vi "Update status--Error.vi"(8 "error in (no error)":errorcluster, 10 "Remove call chain? [Default = False]":bool, 11 "Error message":string) -> (0 "error out":errorcluster)   [LabVIEW 2020, in "status_text_indicator.lvlib"]
uses:
  Status_Text_Indicator.lvlib
  PTRL/String_Control/string_control.lvlib
panel:
  # "Development\ncontrols/indicators useful for development and testing, but which are not outputs of the VI"
  # "Input\nInputs to the VI"
  # "Output\nOutputs of the VI"
  # "Description\n\nBlank VI with error handling case. \n\nSummarize the use of this VI in this space."
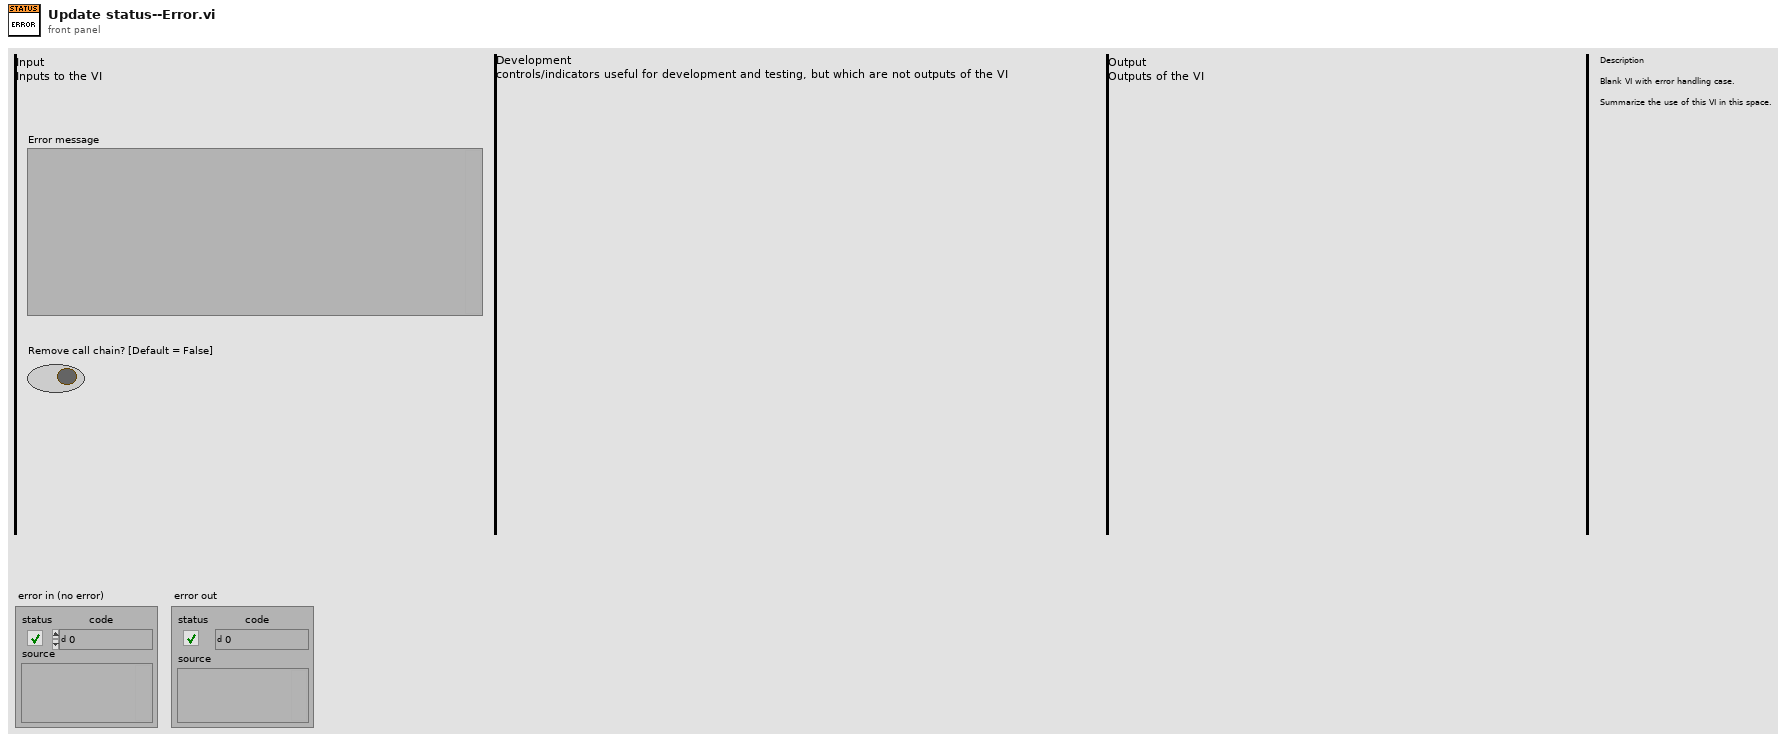
[diagram p1: front panel]
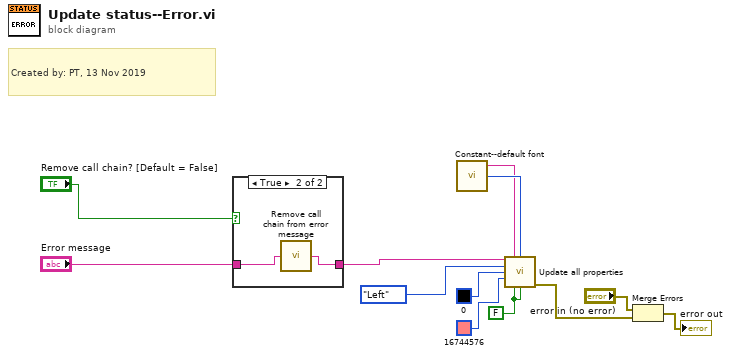
[diagram p0: block diagram]
diagram:
  w9 = FALSE ("Bold? [Default = False]")
  # "Created by: PT, 13 Nov 2019"
  n1 = case shown="True" "Remove call chain? [Default = False]" {
    tunnel: [w13 w14] -> w2
    tunnel: "Error message" -> [w13 w15]
    frame False {
    }
    frame True {
      n2 = call "Remove call chain from error message.vi"("Error message in"=w15) -> ("Error message out (text before call chain)"=w14:string)
    }
  }
  n3 = call "Constant--default font.vi"() -> ("Font size"=w8:u32, "Font name"=w7:string)  [unwired: 1 in]
  n4 = call "Update all properties.vi"("String Value  [Default = \"\" (blank)]"=w2, "Font Name [Default = \"Application Font\"]"=w7, "Font size [Default = 15]"=w8, "Justification [Default = Left]"=enum16{"Left", "Center", "Right"}."Left", "Text Colour [Default=Pure Black=(0,0,0)]"=u32 0 ("Background color"), "Background Colour [Default=Pure White=(255,255,255)]"=u32 16744576 ("Text color"), "Bold? [Default = False]"=w9, "Italic? [Default = False]"=w9) -> ("error out"=w10:errorcluster)  [unwired: 7 in]
  n5 = Merge Errors("error in (no error)", w10) -> (→"error out":errorcluster)
